vi "config_Scope.vi"(0 "instrument handle":refnum<k15>, 1 "trigger source":T1="0" caption="trigger source (Channel 0)", 3 "trigger level":dbl format="%.2f", 5 "Channel":i32, 7 "vertical range":dbl=10.0 format="%.2f", 9 "vertical offset":dbl format="%.4f", 11 "error in":errorcluster, 12 "Frequency(MHz)":dbl, 14 "Time(us)":dbl) -> (4 "instrument handle out":refnum<k15>, 8 "Record length":i32, 10 "Channel out":string, 15 "error out":errorcluster)   [LabVIEW 2016]
uses:
  <instrlib>/niScope/Controls/niScope trigger source.ctl
  <instrlib>/niScope/Controls/niScope vertical coupling.ctl
  <instrlib>/niScope/Controls/niScope trigger slope.ctl
  <instrlib>/niScope/Controls/niScope trigger coupling.ctl
  <instrlib>/niScope/Configure/Trigger/niScope Configure Trigger Edge.vi
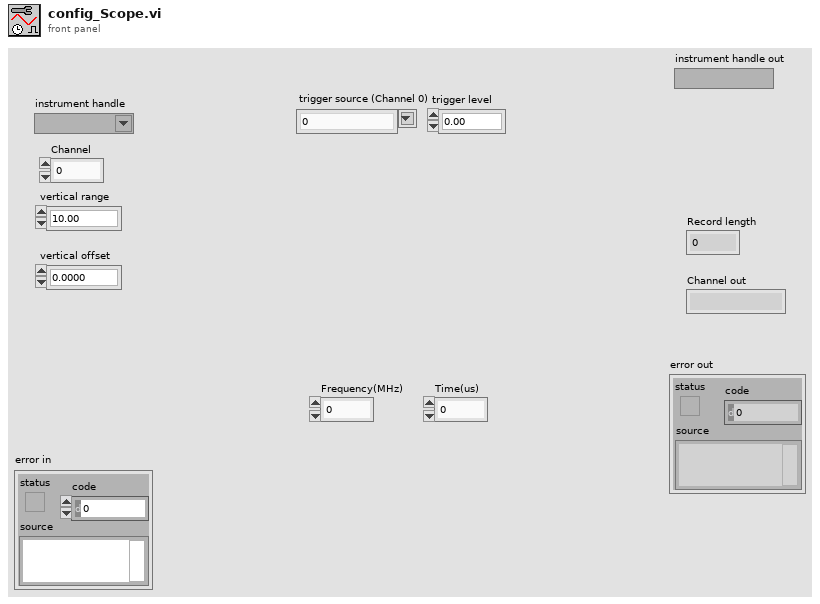
[diagram p1: front panel]
types:
  T1 = typedef "niScope trigger source.ctl" = string
  T2 = typedef "niScope trigger coupling.ctl" = u16
  T3 = typedef "niScope trigger slope.ctl" = i32
  T4 = typedef "niScope vertical coupling.ctl" = i32
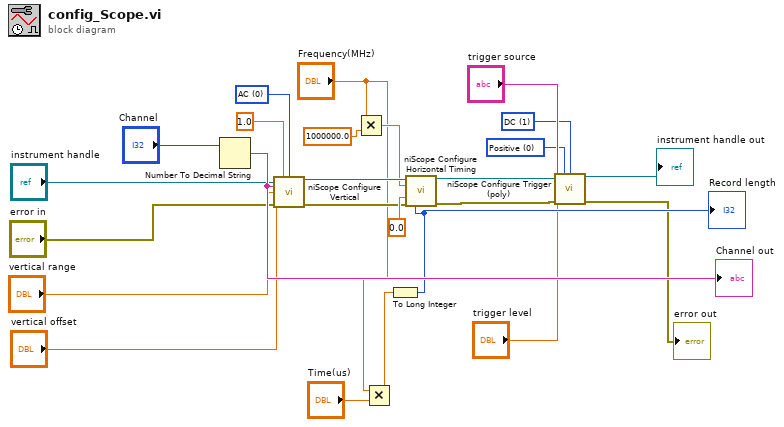
[diagram p0: block diagram]
diagram:
  w1 = T2 1 items=["AC"=0, "DC"=1, "HF Reject"=3, "LF Reject"=4, "AC Plus HF Reject"=1001] ("trigger coupling")
  w2 = T3 0 items=["Positive", "Negative"] ("trigger slope")
  w22 = T4 0 items=["AC", "DC", "Ground"] ("vertical coupling")
  n1 = Number To Decimal String(number="Channel") -> (decimal integer string=w24:string)  [unwired: 1 in]
  "Channel out" <- w24
  n2 = call <instrlib>:"niScope Configure Vertical.vi"("instrument handle"="instrument handle", "probe attenuation"=1.0, "vertical coupling"=w22, "channels"=w24, "vertical range"="vertical range", "vertical offset"="vertical offset", "error in"="error in") -> ("instrument handle out"=w16:refnum<k15>, "error out"=w15:errorcluster)  [unwired: 7 in]
  n3 = Multiply(x="Frequency(MHz)", y=1000000.0 ("min sample rate")) -> (x*y=w14:dbl)
  n4 = Multiply(x="Frequency(MHz)", y="Time(us)") -> (x*y=w12:dbl)
  n5 = To Long Integer(number=w12) -> (32bit integer=w9:i32)
  "Record length" <- w9
  n6 = call <instrlib>:"niScope Configure Horizontal Timing.vi"("instrument handle"=w16, "min sample rate"=w14, "reference position"=0.0, "error in"=w15, "min record length"=w9) -> ("instrument handle out"=w8:refnum<k15>, "error out"=w7:errorcluster)  [unwired: 9 in]
  n7 = call-poly <instrlib>:"niScope Configure Trigger (poly).vi"("instrument handle"=w8, "trigger slope"=w2, "trigger coupling"=w1, "trigger source"="trigger source", "trigger level"="trigger level", "error in"=w7) -> ("instrument handle out"=→"instrument handle out":refnum<k15>, "error out"=→"error out":errorcluster)  [unwired: 8 in]
